vi "Channel Inputs.vi"(0 "Data Notifier":refnum<notifier>, 11 "error in":errorcluster={"status"=TRUE, "code"=0, "source"=""}) -> (3 "BangBang\nArm out":bool, 4 "Data Notifier out":refnum<notifier>, 6 "Actuation Array":bool[](array[boolean]), 10 "Auto-sequence":bool, 14 "Abort":bool, 15 "error out":errorcluster)   [LabVIEW 2024]
uses:
  78c51032-1941-47d2-9962-ba45e907be92.vi
  <vilib>/ErrorRing/Error Ring.xnode
  <vilib>/Utility/error.llb/Error Cluster From Error Code.vi
  support/Control/Array Data Constant.ctl
panel:
  in  "Prop Test":T1(array[cluster])=[{"Valve Label"="Fuel Iso", "Valve Index"=10, "Talkback Index"=9, "Actuate?"=TRUE, "Timeout"=10.0}, {"Valve Label"="LOX Iso", "Valve Index"=3, "Talkback Index"=3, "Actuate?"=TRUE, "Timeout"=10.0}, {"Valve Label"="Fuel Main", "Valve Index"=11, "Talkback Index"=10, "Actuate?"=TRUE, "Timeout"=10.0}, {"Valve Label"="LOX Main", "Valve Index"=4, "Talkback Index"=4, "Actuate?"=TRUE, "Timeout"=10.0}, {"Valve Label"="LOX Bleed", "Valve Index"=5, "Talkback Index"=5, "Actuate?"=TRUE, "Timeout"=10.0}]
  in  "NonProp Test":T1(array[cluster])=[{"Valve Label"="LOX Press", "Valve Index"=0, "Talkback Index"=0, "Actuate?"=TRUE, "Timeout"=24.0}, {"Valve Label"="Fuel Press", "Valve Index"=7, "Talkback Index"=6, "Actuate?"=TRUE, "Timeout"=24.0}, {"Valve Label"="LOX Vent", "Valve Index"=2, "Talkback Index"=2, "Actuate?"=TRUE, "Timeout"=4.0}, {"Valve Label"="Fuel Vent", "Valve Index"=9, "Talkback Index"=8, "Actuate?"=TRUE, "Timeout"=4.0}, {"Valve Label"="Fuel Purge", "Valve Index"=8, "Talkback Index"=7, "Actuate?"=TRUE, "Timeout"=2.0}, {"Valve Label"="LOX Purge", "Valve Index"=1, "Talkback Index"=1, "Actuate?"=TRUE, "Timeout"=2.0}, {"Valve Label"="Fuel Iso", "Valve Index"=10, "Talkback Index"=9, "Actuate?"=FALSE, "Timeout"=2.0}, {"Valve Label"="LOX Iso", "Valve Index"=3, "Talkback Index"=3, "Actuate?"=FALSE, "Timeout"=2.0}, {"Valve Label"="Fuel Main", "Valve Index"=11, "Talkback Index"=10, "Actuate?"=FALSE, "Timeout"=2.0}, {"Valve Label"="LOX Main", "Valve Index"=4, "Talkback Index"=4, "Actuate?"=FALSE, "Timeout"=2.0}, {"Valve Label"="LOX Bleed", "Valve Index"=5, "Talkback Index"=5, "Actuate?"=FALSE, "Timeout"=2.0}]
  in  "BangBang\nEnable":bool
  out "Time":dbl
  out "Actuate":bool caption="Should\nActuate?"
  out "LED 18":bool
  out "LED 17":bool
  out "LED 16":bool
  out "LED 15":bool
  out "LED 14":bool
  out "LED 13":bool
  out "LED 12":bool
  out "LED 11":bool
  out "LED 10":bool
  out "LED 9":bool
  out "LED 8":bool
  out "LED 7":bool
  out "LED 6":bool
  out "LED 5":bool
  out "LED 4":bool
  out "LED 3":bool
  out "LED 2":bool
  out "LED 1":bool
  out "Actuation Check":string
  in  "Actuation Check":bool caption="TC3\nActuation\nCheck"
  in  "Abort":bool
  in  "Switch 18":bool
  in  "Switch 17":bool
  in  "AutoSeq":bool
  in  "PropFlow":bool
  in  "Switch 16":bool
  in  "Switch 15":bool caption="LOX\nLoad"
  in  "Switch 14":bool caption="LOX\nBleed"
  in  "Switch 13":bool caption="LOX\nMain"
  in  "Switch 12":bool caption="LOX\nIso"
  in  "Switch 11":bool caption="LOX\nVent"
  in  "Switch 10":bool caption="LOX\nPurge"
  in  "Switch 9":bool caption="LOX\nPress"
  in  "Switch 8":bool
  in  "Switch 7":bool
  in  "Switch 6":bool
  in  "Switch 5":bool caption="Fuel\nMain"
  in  "Switch 4":bool caption="Fuel\nIso"
  in  "Switch 3":bool caption="Fuel\nVent"
  in  "Switch 2":bool caption="Fuel\nPurge"
  in  "Switch 1":bool caption="Fuel\nPress"
  in  "Software\nSwitch":bool
  out "Prop Flow":bool
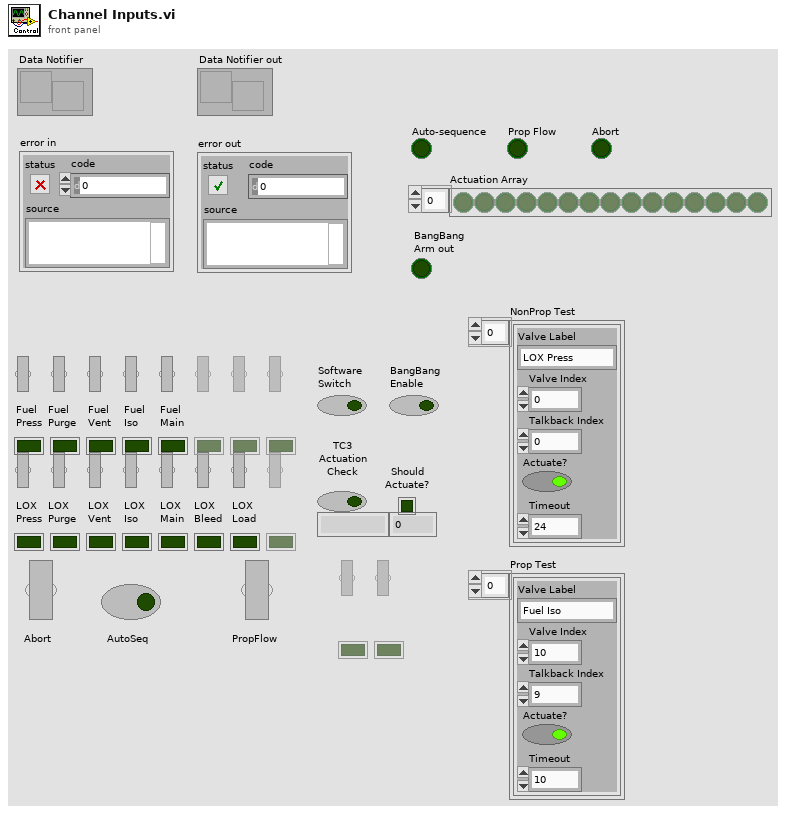
[diagram p1: front panel]
types:
  T1 = cluster{"Valve Label":string, "Valve Index":i32, "Talkback Index":i32, "Actuate?":bool, "Timeout":dbl}[]
  T2 = typedef "Array Data Constant.ctl" = cluster{"AI":dbl[], "TC":dbl[], "BC":dbl[], "DI":dbl[], "t (UTC)":dbl}
  T3 = cluster{"[0]":bool, "[1]":bool, "[2]":bool, "[3]":bool, "[4]":bool, "[5]":bool, "[6]":bool, "[7]":bool, "[8]":bool, "[9]":bool, "[10]":bool, "[11]":bool, "[12]":bool, "[13]":bool, "[14]":bool, "[15]":bool}
  T4 = cluster{"Valve Label":string, "Valve Index":i32, "Talkback Index":i32, "Actuate?":bool, "Timeout":dbl}
  T5 = cluster{"Switch 9":bool, "Switch 10":bool, "Switch 11":bool, bool, bool, bool, bool, "Switch 1":bool, "Switch 2":bool, "Switch 3":bool, bool, bool, bool, bool, bool, bool, bool, bool, bool, bool}
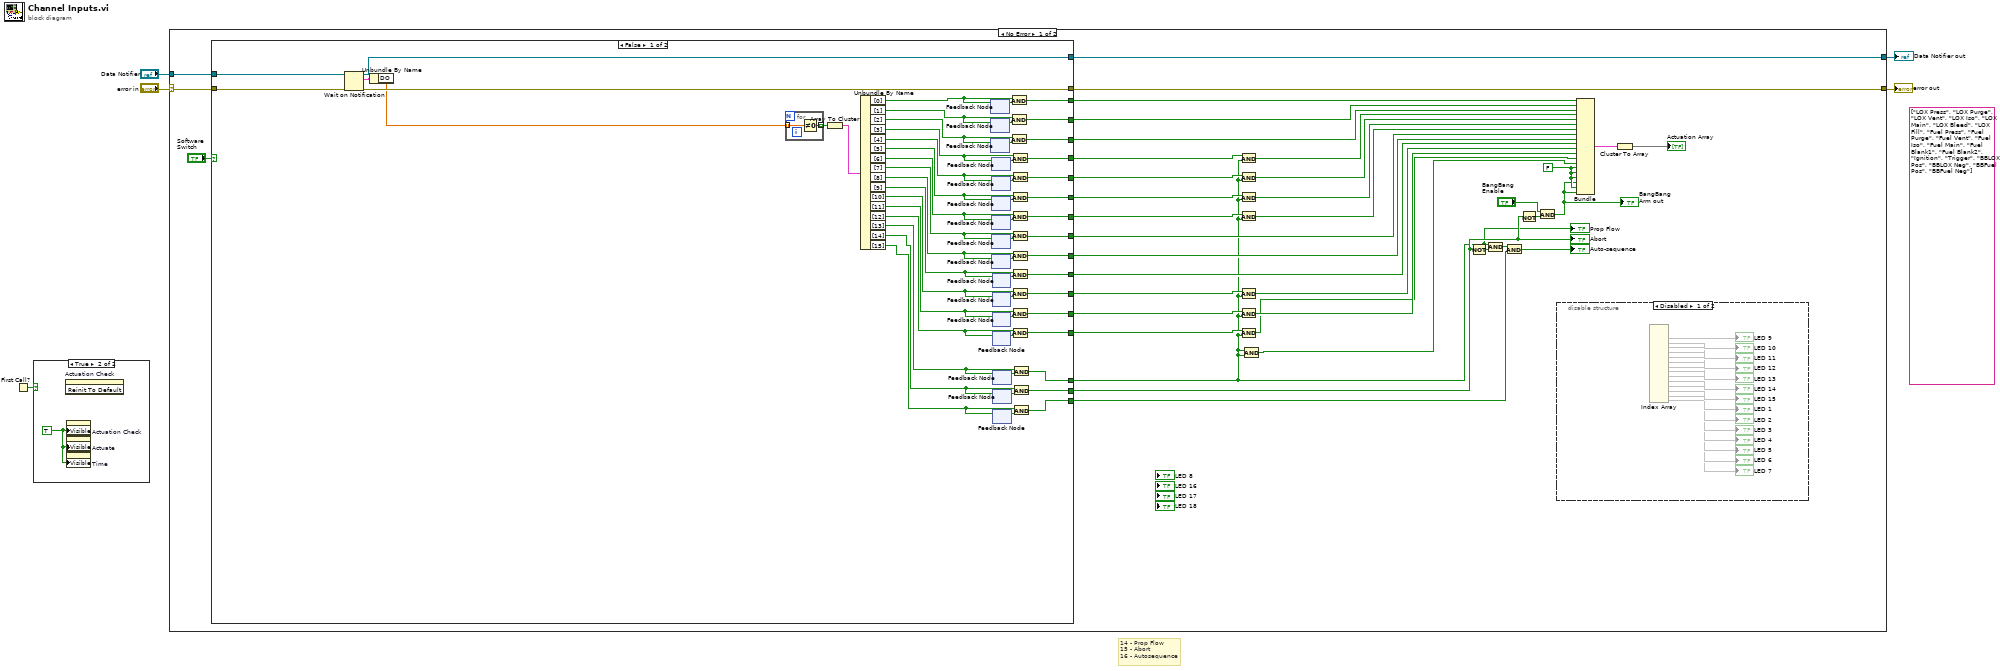
[diagram p0: block diagram]
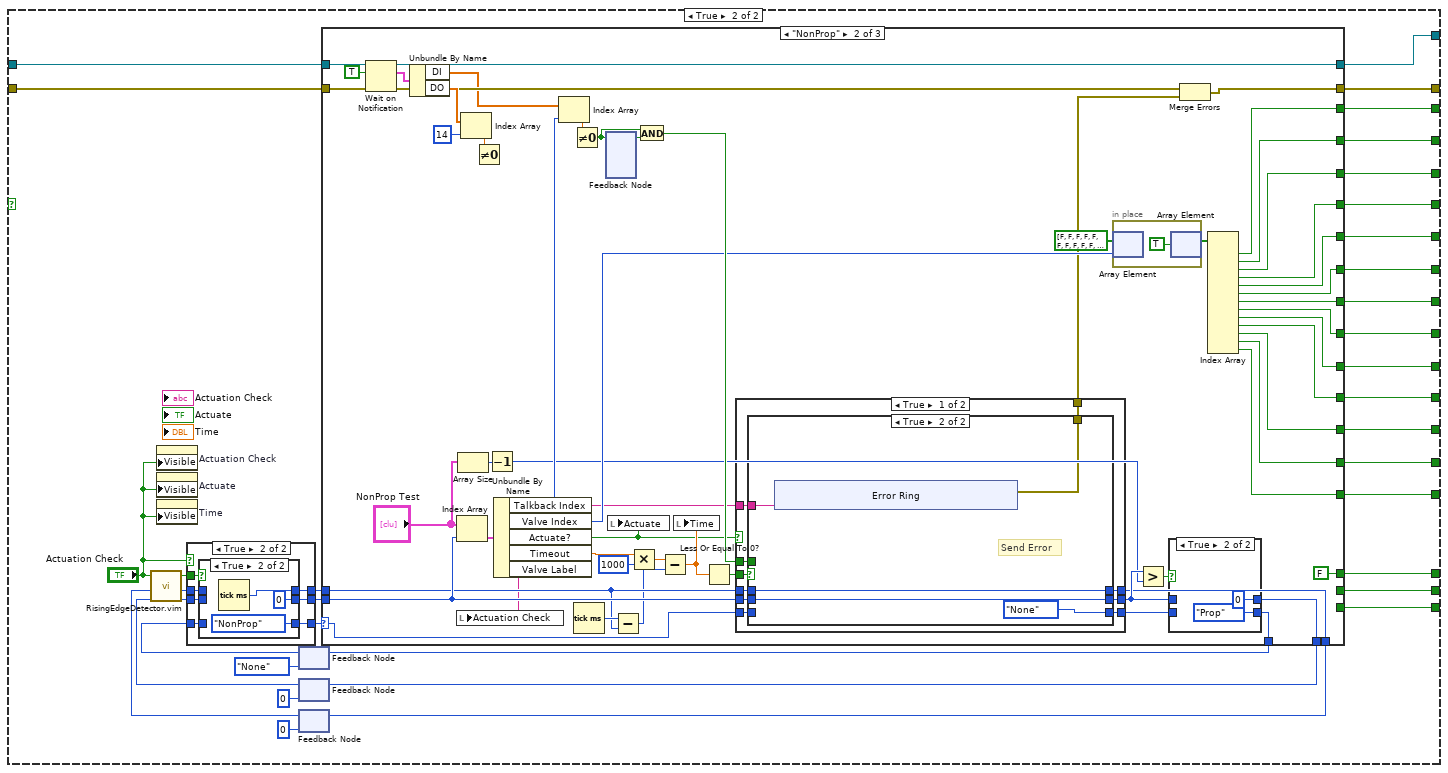
[diagram p4: hidden frame]
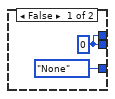
[diagram p5: hidden frame]
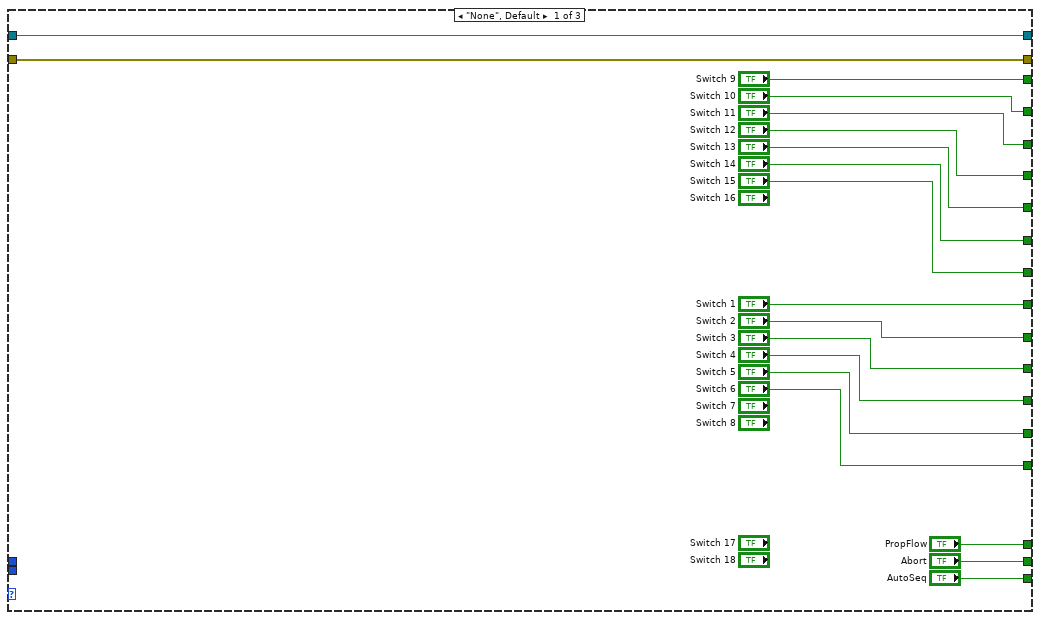
[diagram p7: hidden frame]
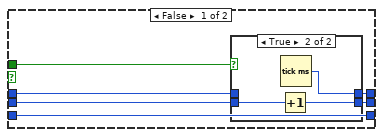
[diagram p9: hidden frame]
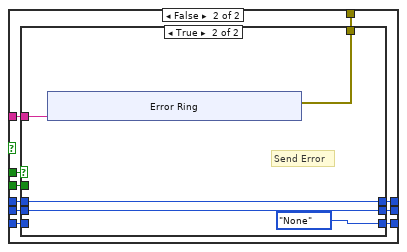
[diagram p11: hidden frame]
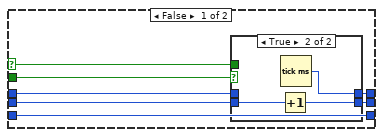
[diagram p12: hidden frame]
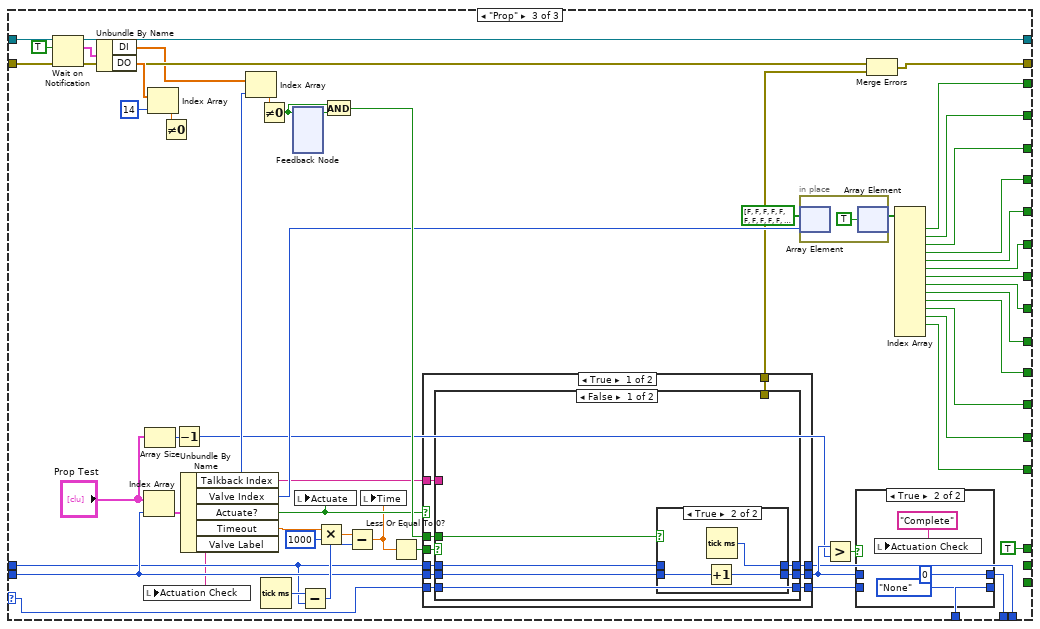
[diagram p14: hidden frame]
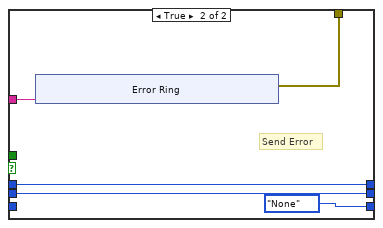
[diagram p17: hidden frame]
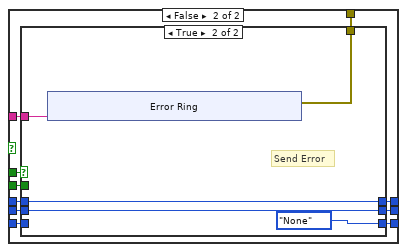
[diagram p18: hidden frame]
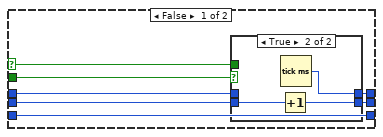
[diagram p19: hidden frame]
diagram:
  (unwired) string[] ["LOX Press", "LOX Purge", "LOX Vent", "LOX Iso", "LOX Main", "LOX Bleed", "LOX Fill", "Fuel Press", "Fuel Purge", "Fuel Vent", "Fuel Iso", "Fuel Main", "Fuel Blank1", "Fuel Blank2", "Ignition", "Trigger", "BBLOX Pos", "BBLOX Neg", "BBFuel Pos", "BBFuel Neg"]
  # "14 - Prop Flow\n15 - Abort\n16 - Autosequence"
  n1 = First Call?() -> (First Call?: T/F=w1:bool)
  n2 = case shown="True" w1 {
    frame False {
    }
    frame True {
      w6 = TRUE ("Visible")
      n3 = invoke on="Actuation Check" class="Bool (strict)" method="Reinit To Default"() -> ()  [unwired: 3 in, 3 out]
      n4 = property on="Actuation Check" class="Str"("Visible"=w6) -> ()  [unwired: 2 in, 2 out]
      n5 = property on="Actuate" class="Bool (strict)"("Visible"=w6) -> ()  [unwired: 2 in, 2 out]
      n6 = property on="Time" class="DigNum (strict)"("Visible"=w6) -> ()  [unwired: 2 in, 2 out]
    }
  }
  n7 = case shown="No Error" "error in" {
    selector: "error in" -> [w44 w442]
    tunnel: [w43 w442] -> w4
    tunnel: "Data Notifier" -> [w36 w441]
    tunnel: [w23 w441] -> w2
    frame No Error {
      w22 = FALSE
      n8 = case shown="False" "Software\nSwitch" {
        tunnel: w44 -> [w69 w124]
        tunnel: [w68 w123] -> w43
        tunnel: [w114 w149] -> w7
        tunnel: [w93 w148] -> w35
        tunnel: [w92 w141] -> w34
        tunnel: [w91 w140] -> w33
        tunnel: [w90 w139] -> w32
        tunnel: [w89 w138] -> w31
        tunnel: [w88 w137] -> w30
        tunnel: [w87 w150] -> w38
        tunnel: [w86 w135] -> w18
        tunnel: [w75 w136] -> w29
        tunnel: [w74 w147] -> w28
        tunnel: [w73 w146] -> w27
        tunnel: [w72 w145] -> w26
        tunnel: [w71 w144] -> w16
        tunnel: [w70 w143] -> w17
        tunnel: [w59 w142] -> w25
        tunnel: w36 -> [w67 w134]
        tunnel: [w66 w133] -> w23
        frame False {
          n9 = Wait on Notification(notifier=w67, error in (no error)=w69) -> (notifier out=w66:refnum<notifier>, notification=w65:T2, error out=w68:errorcluster)  [unwired: 2 in, 1 out]
          n10 = Unbundle By Name(w65) -> ("DO"=w64:dbl[])
          n11 = for {
            tunnel: w64 -> [w115] mode=indexing
            tunnel: [w116] -> w63 mode=indexing
            n12 = Not Equal To 0?(x=w115) -> (x != 0?=w116:bool)
          }
          n13 = Array To Cluster(array=w63) -> (cluster=w113:T3)
          n14 = Unbundle By Name(w113) -> ("[0]"=w96:bool, "[1]"=w95:bool, "[2]"=w94:bool, "[3]"=w85:bool, "[4]"=w84:bool, "[5]"=w83:bool, "[6]"=w82:bool, "[7]"=w81:bool, "[8]"=w80:bool, "[9]"=w79:bool, "[10]"=w78:bool, "[11]"=w77:bool, "[12]"=w76:bool, "[13]"=w62:bool, "[14]"=w61:bool, "[15]"=w60:bool)
          n15 = feedback #1() -> (w112:bool)  [unwired: 1 in]
          n16 = feedback-in #1(w96) -> ()
          n17 = feedback #2() -> (w111:bool)  [unwired: 1 in]
          n18 = feedback-in #2(w95) -> ()
          n19 = feedback #3() -> (w110:bool)  [unwired: 1 in]
          n20 = feedback-in #3(w94) -> ()
          n21 = feedback #4() -> (w109:bool)  [unwired: 1 in]
          n22 = feedback-in #4(w85) -> ()
          n23 = feedback #5() -> (w108:bool)  [unwired: 1 in]
          n24 = feedback-in #5(w84) -> ()
          n25 = feedback #6() -> (w107:bool)  [unwired: 1 in]
          n26 = feedback-in #6(w83) -> ()
          n27 = feedback #7() -> (w106:bool)  [unwired: 1 in]
          n28 = feedback-in #7(w82) -> ()
          n29 = feedback #8() -> (w105:bool)  [unwired: 1 in]
          n30 = feedback-in #8(w81) -> ()
          n31 = feedback #9() -> (w104:bool)  [unwired: 1 in]
          n32 = feedback-in #9(w80) -> ()
          n33 = feedback #10() -> (w103:bool)  [unwired: 1 in]
          n34 = feedback-in #10(w79) -> ()
          n35 = feedback #11() -> (w102:bool)  [unwired: 1 in]
          n36 = feedback-in #11(w78) -> ()
          n37 = feedback #12() -> (w101:bool)  [unwired: 1 in]
          n38 = feedback-in #12(w77) -> ()
          n39 = feedback #13() -> (w100:bool)  [unwired: 1 in]
          n40 = feedback-in #13(w76) -> ()
          n41 = feedback #14() -> (w99:bool)  [unwired: 1 in]
          n42 = feedback-in #14(w62) -> ()
          n43 = feedback #15() -> (w98:bool)  [unwired: 1 in]
          n44 = feedback-in #15(w61) -> ()
          n45 = feedback #16() -> (w97:bool)  [unwired: 1 in]
          n46 = feedback-in #16(w60) -> ()
          n47 = And(x=w96, y=w112) -> (x .and. y?=w93:bool)
          n48 = And(x=w95, y=w111) -> (x .and. y?=w92:bool)
          n49 = And(x=w94, y=w110) -> (x .and. y?=w91:bool)
          n50 = And(x=w85, y=w109) -> (x .and. y?=w90:bool)
          n51 = And(x=w84, y=w108) -> (x .and. y?=w89:bool)
          n52 = And(x=w83, y=w107) -> (x .and. y?=w88:bool)
          n53 = And(x=w82, y=w106) -> (x .and. y?=w75:bool)
          n54 = And(x=w81, y=w105) -> (x .and. y?=w74:bool)
          n55 = And(x=w80, y=w104) -> (x .and. y?=w73:bool)
          n56 = And(x=w79, y=w103) -> (x .and. y?=w72:bool)
          n57 = And(x=w78, y=w102) -> (x .and. y?=w71:bool)
          n58 = And(x=w77, y=w101) -> (x .and. y?=w70:bool)
          n59 = And(x=w76, y=w100) -> (x .and. y?=w59:bool)
          n60 = And(x=w62, y=w99) -> (x .and. y?=w114:bool)
          n61 = And(x=w61, y=w98) -> (x .and. y?=w86:bool)
          n62 = And(x=w60, y=w97) -> (x .and. y?=w87:bool)
        }
        frame True {
          n63 = call "RisingEdgeDetector.vim"("Data"="Actuation Check") -> ("Edge?"=w118:bool)  [unwired: 4 in]
          n64 = property on="Actuation Check" class="Str"("Visible"="Actuation Check") -> ()  [unwired: 2 in, 2 out]
          n65 = property on="Actuate" class="Bool (strict)"("Visible"="Actuation Check") -> ()  [unwired: 2 in, 2 out]
          n66 = property on="Time" class="DigNum (strict)"("Visible"="Actuation Check") -> ()  [unwired: 2 in, 2 out]
          n67 = feedback #17(enum16{"None", "NonProp", "Prop"}."None") -> (w131:enum16{"None", "NonProp", "Prop"})
          n68 = feedback #18(u8 0) -> (w127:u8)
          n69 = feedback #19(u32 0) -> (w121:u32)
          n70 = case shown="True" "Actuation Check" {
            tunnel: w131 -> [_ w159]
            tunnel: [enum16{"None", "NonProp", "Prop"}."None" w158] -> w130
            tunnel: w127 -> [_ w157]
            tunnel: [w151 w156] -> w126
            tunnel: w121 -> [_ w155]
            tunnel: [w151 w154] -> w119
            tunnel: w118 -> [_ w153]
            frame False {
              w151 = u8 0
            }
            frame True {
              n71 = case shown="True" w153 {
                tunnel: w159 -> [w162 _]
                tunnel: [w162 enum16{"None", "NonProp", "Prop"}."NonProp"] -> w158
                tunnel: w157 -> [w161 _]
                tunnel: [w161 u8 0] -> w156
                tunnel: [w160 w163] -> w154
                tunnel: w155 -> [w160 _]
                frame False {
                }
                frame True {
                  n72 = Tick Count (ms)() -> (millisecond timer value=w163:u32)
                }
              }
            }
          }
          n73 = case shown="\"NonProp\"" w130 {
            selector: w130 -> [_ w201 w328]
            tunnel: ["AutoSeq" _ _] -> w150
            tunnel: ["PropFlow" FALSE ("PropFlow") TRUE ("PropFlow")] -> w149
            tunnel: ["Switch 9" w227 w355] -> w148
            tunnel: ["Switch 1" w220 w348] -> w147
            tunnel: ["Switch 2" w219 w347] -> w146
            tunnel: ["Switch 3" w218 w346] -> w145
            tunnel: ["Switch 4" w217 w345] -> w144
            tunnel: ["Switch 5" w216 w344] -> w143
            tunnel: ["Switch 6" w215 w343] -> w142
            tunnel: ["Switch 10" w226 w354] -> w141
            tunnel: ["Switch 11" w225 w353] -> w140
            tunnel: ["Switch 12" w224 w352] -> w139
            tunnel: ["Switch 13" w223 w351] -> w138
            tunnel: ["Switch 14" w222 w350] -> w137
            tunnel: ["Switch 15" w221 w349] -> w136
            tunnel: ["Abort" _ _] -> w135
            tunnel: w134 -> [w168 w237 w365]
            tunnel: [w168 w235 w363] -> w133
            tunnel: [_ w196 w323] -> w129
            tunnel: [_ w194 w321] -> w128
            tunnel: w126 -> [_ w208 w335]
            tunnel: w124 -> [w167 w236 w364]
            tunnel: [w167 w203 w330] -> w123
            tunnel: [_ w192 w319] -> w120
            tunnel: w119 -> [_ w193 w320]
            frame "None", Default {
            }
            frame "NonProp" {
              n74 = Wait on Notification(notifier=w237, ignore previous (F)=TRUE, error in (no error)=w236) -> (notifier out=w235:refnum<notifier>, notification=w234:T2, error out=w204:errorcluster)  [unwired: 1 in, 1 out]
              n75 = Unbundle By Name(w234) -> ("DI"=w188:dbl[], "DO"=w230:dbl[])
              n76 = Index Array(array="NonProp Test", index=w208) -> (element=w239:T4)
              n77 = Array Size(array="NonProp Test") -> (size(s)=w199:i32)
              n78 = Index Array(array=w230, index=14) -> (element=w229:dbl)
              n79 = Not Equal To 0?(x=w229) -> ()  [unwired: 1 out]
              n80 = Decrement(x=w199) -> (x-1=w190:i32)
              n81 = Unbundle By Name(w239) -> ("Talkback Index"=w212:i32, "Valve Index"=w205:i32, "Actuate?"=w184:bool, "Timeout"=w210:dbl, "Valve Label"=w189:string)
              n82 = local write "Actuation Check"(w189) -> ()
              n83 = Index Array(array=w188, index=w212) -> (element=w228:dbl)
              n84 = Not Equal To 0?(x=w228) -> (x != 0?=w232:bool)
              n85 = Tick Count (ms)() -> (millisecond timer value=w209:u32)
              n86 = feedback-in #20(w232) -> ()
              n87 = feedback #20() -> (w233:bool)  [unwired: 1 in]
              n88 = local write "Actuate"(w184) -> ()
              n89 = Subtract(x=w209, y=w193) -> (x-y=w187:u32)
              n90 = Multiply(x=w210, y=u32 1000 ("x")) -> (x*y=w186:dbl)
              n91 = And(x=w232, y=w233) -> (x .and. y?=w206:bool)
              n92 = Subtract(x=w186, y=w187) -> (x-y=w185:dbl)
              n93 = local write "Time"(w185) -> ()
              n94 = Less Or Equal To 0?(x=w185) -> (x <= 0?=w207:bool)
              n95 = case shown="True" w184 {
                tunnel: w208 -> [w252 w285]
                tunnel: [w251 w284] -> w195
                tunnel: w207 -> [w253 w286]
                tunnel: w206 -> [w250 w283]
                tunnel: [w249 w282] -> w202
                tunnel: [w248 w281] -> w197
                tunnel: w201 -> [w247 w280]
                tunnel: w193 -> [w246 w279]
                tunnel: [w245 w278] -> w192
                tunnel: w189 -> [w244 w277]
                frame True {
                  n96 = case shown="True" w253 {
                    tunnel: w252 -> [w258 w269]
                    tunnel: [w257 w269] -> w251
                    tunnel: w250 -> [w259 _]
                    tunnel: [_ w266] -> w249
                    tunnel: [w256 enum16{"None", "NonProp", "Prop"}."None"] -> w248
                    tunnel: w247 -> [w256 _]
                    tunnel: w246 -> [w255 w267]
                    tunnel: [w254 w267] -> w245
                    tunnel: w244 -> [_ w265]
                    frame False {
                      n97 = case shown="True" w259 {
                        tunnel: w258 -> [w261 w264]
                        tunnel: [w261 w263] -> w257
                        tunnel: w255 -> [w260 _]
                        tunnel: [w260 w262] -> w254
                        frame False {
                        }
                        frame True {
                          n98 = Increment(x=w264) -> (x+1=w263:u8)
                          n99 = Tick Count (ms)() -> (millisecond timer value=w262:u32)
                        }
                      }
                    }
                    frame True {
                      # "Send Error"
                      n100 = xnode "Error Ring"("parameter 0"=w265) -> ("error out"=w266:errorcluster)
                    }
                  }
                }
                frame False {
                  n101 = case shown="True" w283 {
                    selector: w283 -> [w293 _]
                    tunnel: w285 -> [w292 w303]
                    tunnel: [w291 w303] -> w284
                    tunnel: [_ w300] -> w282
                    tunnel: [w290 enum16{"None", "NonProp", "Prop"}."None"] -> w281
                    tunnel: w280 -> [w290 _]
                    tunnel: w286 -> [w289 _]
                    tunnel: w279 -> [w288 w301]
                    tunnel: [w287 w301] -> w278
                    tunnel: w277 -> [_ w299]
                    frame False {
                      n102 = case shown="True" w289 {
                        tunnel: w292 -> [w295 w298]
                        tunnel: [w295 w297] -> w291
                        tunnel: w293 -> [_ _]
                        tunnel: w288 -> [w294 _]
                        tunnel: [w294 w296] -> w287
                        frame False {
                        }
                        frame True {
                          n103 = Increment(x=w298) -> (x+1=w297:u8)
                          n104 = Tick Count (ms)() -> (millisecond timer value=w296:u32)
                        }
                      }
                    }
                    frame True {
                      # "Send Error"
                      n105 = xnode "Error Ring"("parameter 0"=w299) -> ("error out"=w300:errorcluster)
                    }
                  }
                }
              }
              n106 = in-place {
                n107 = in-place-array #21(bool[] [FALSE, FALSE, FALSE, FALSE, FALSE, FALSE, FALSE, FALSE, FALSE, FALSE, FALSE, FALSE, FALSE, FALSE, FALSE, FALSE, FALSE, FALSE, FALSE, FALSE, FALSE], w205) -> ()  [unwired: 1 out]
                n108 = in-place-array #21(TRUE ("element")) -> (w213:bool[])  [unwired: 1 out]
              }
              n109 = Greater?(x=w195, y=w190) -> (0:w198:bool)
              n110 = case shown="True" w198 {
                tunnel: w197 -> [w240 _]
                tunnel: [w240 enum16{"None", "NonProp", "Prop"}."Prop"] -> w196
                tunnel: w195 -> [w241 _]
                tunnel: [w241 u8 0] -> w194
                frame False {
                }
                frame True {
                }
              }
              n111 = Merge Errors(w204, w202) -> (w203:errorcluster)
              n112 = Index Array(array=w213) -> (element #1=w227:bool, element #2=w226:bool, element #3=w225:bool, element #4=w224:bool, element #5=w223:bool, element #6=w222:bool, element #7=w221:bool, element #8=w220:bool, element #9=w219:bool, element #10=w218:bool, element #11=w217:bool, element #12=w216:bool, element #13=w215:bool)  [unwired: 13 in]
            }
            frame "Prop" {
              n113 = Wait on Notification(notifier=w365, ignore previous (F)=TRUE, error in (no error)=w364) -> (notifier out=w363:refnum<notifier>, notification=w362:T2, error out=w331:errorcluster)  [unwired: 1 in, 1 out]
              n114 = Unbundle By Name(w362) -> ("DI"=w315:dbl[], "DO"=w358:dbl[])
              n115 = Index Array(array="Prop Test", index=w335) -> (element=w367:T4)
              n116 = Array Size(array="Prop Test") -> (size(s)=w326:i32)
              n117 = Index Array(array=w358, index=14) -> (element=w357:dbl)
              n118 = Not Equal To 0?(x=w357) -> ()  [unwired: 1 out]
              n119 = Decrement(x=w326) -> (x-1=w317:i32)
              n120 = Unbundle By Name(w367) -> ("Talkback Index"=w340:i32, "Valve Index"=w332:i32, "Actuate?"=w314:bool, "Timeout"=w338:dbl, "Valve Label"=w316:string)
              n121 = local write "Actuation Check"(w316) -> ()
              n122 = Index Array(array=w315, index=w340) -> (element=w356:dbl)
              n123 = Not Equal To 0?(x=w356) -> (x != 0?=w360:bool)
              n124 = Tick Count (ms)() -> (millisecond timer value=w337:u32)
              n125 = feedback-in #22(w360) -> ()
              n126 = feedback #22() -> (w361:bool)  [unwired: 1 in]
              n127 = local write "Actuate"(w314) -> ()
              n128 = Subtract(x=w337, y=w320) -> (x-y=w336:u32)
              n129 = Multiply(x=w338, y=u32 1000 ("x")) -> (x*y=w313:dbl)
              n130 = And(x=w360, y=w361) -> (x .and. y?=w333:bool)
              n131 = Subtract(x=w313, y=w336) -> (x-y=w312:dbl)
              n132 = local write "Time"(w312) -> ()
              n133 = Less Or Equal To 0?(x=w312) -> (x <= 0?=w334:bool)
              n134 = case shown="True" w314 {
                tunnel: w335 -> [w381 w414]
                tunnel: [w380 w413] -> w322
                tunnel: w334 -> [w382 w415]
                tunnel: w333 -> [w379 w412]
                tunnel: [w378 w411] -> w329
                tunnel: [w377 w410] -> w324
                tunnel: w328 -> [w376 w409]
                tunnel: w320 -> [w375 w408]
                tunnel: [w374 w407] -> w319
                tunnel: w316 -> [w373 w406]
                frame True {
                  n135 = case shown="False" w382 {
                    tunnel: w381 -> [w387 w398]
                    tunnel: [w386 w398] -> w380
                    tunnel: w379 -> [w388 _]
                    tunnel: [_ w395] -> w378
                    tunnel: [w385 enum16{"None", "NonProp", "Prop"}."None"] -> w377
                    tunnel: w376 -> [w385 _]
                    tunnel: w375 -> [w384 w396]
                    tunnel: [w383 w396] -> w374
                    tunnel: w373 -> [_ w394]
                    frame False {
                      n136 = case shown="True" w388 {
                        tunnel: w387 -> [w390 w393]
                        tunnel: [w390 w392] -> w386
                        tunnel: w384 -> [w389 _]
                        tunnel: [w389 w391] -> w383
                        frame False {
                        }
                        frame True {
                          n137 = Increment(x=w393) -> (x+1=w392:u8)
                          n138 = Tick Count (ms)() -> (millisecond timer value=w391:u32)
                        }
                      }
                    }
                    frame True {
                      # "Send Error"
                      n139 = xnode "Error Ring"("parameter 0"=w394) -> ("error out"=w395:errorcluster)
                    }
                  }
                }
                frame False {
                  n140 = case shown="True" w412 {
                    selector: w412 -> [w422 _]
                    tunnel: w414 -> [w421 w432]
                    tunnel: [w420 w432] -> w413
                    tunnel: [_ w429] -> w411
                    tunnel: [w419 enum16{"None", "NonProp", "Prop"}."None"] -> w410
                    tunnel: w409 -> [w419 _]
                    tunnel: w415 -> [w418 _]
                    tunnel: w408 -> [w417 w430]
                    tunnel: [w416 w430] -> w407
                    tunnel: w406 -> [_ w428]
                    frame False {
                      n141 = case shown="True" w418 {
                        tunnel: w421 -> [w424 w427]
                        tunnel: [w424 w426] -> w420
                        tunnel: w422 -> [_ _]
                        tunnel: w417 -> [w423 _]
                        tunnel: [w423 w425] -> w416
                        frame False {
                        }
                        frame True {
                          n142 = Increment(x=w427) -> (x+1=w426:u8)
                          n143 = Tick Count (ms)() -> (millisecond timer value=w425:u32)
                        }
                      }
                    }
                    frame True {
                      # "Send Error"
                      n144 = xnode "Error Ring"("parameter 0"=w428) -> ("error out"=w429:errorcluster)
                    }
                  }
                }
              }
              n145 = in-place {
                n146 = in-place-array #23(bool[] [FALSE, FALSE, FALSE, FALSE, FALSE, FALSE, FALSE, FALSE, FALSE, FALSE, FALSE, FALSE, FALSE, FALSE, FALSE, FALSE, FALSE, FALSE, FALSE, FALSE, FALSE], w332) -> ()  [unwired: 1 out]
                n147 = in-place-array #23(TRUE ("element")) -> (w341:bool[])  [unwired: 1 out]
              }
              n148 = Greater?(x=w322, y=w317) -> (0:w325:bool)
              n149 = case shown="True" w325 {
                tunnel: w324 -> [w368 _]
                tunnel: [w368 enum16{"None", "NonProp", "Prop"}."None"] -> w323
                tunnel: w322 -> [w369 _]
                tunnel: [w369 u8 0] -> w321
                frame False {
                }
                frame True {
                  n150 = local write "Actuation Check"("Complete") -> ()
                }
              }
              n151 = Merge Errors(w331, w329) -> (w330:errorcluster)
              n152 = Index Array(array=w341) -> (element #1=w355:bool, element #2=w354:bool, element #3=w353:bool, element #4=w352:bool, element #5=w351:bool, element #6=w350:bool, element #7=w349:bool, element #8=w348:bool, element #9=w347:bool, element #10=w346:bool, element #11=w345:bool, element #12=w344:bool, element #13=w343:bool)  [unwired: 14 in, 1 out]
            }
          }
          n153 = feedback-in #17(w129) -> ()
          n154 = feedback-in #18(w128) -> ()
          n155 = feedback-in #19(w120) -> ()
        }
      }
      "Prop Flow" <- w7
      "Abort" <- w18
      n156 = And(x=w32, y=w7) -> (x .and. y?=w15:bool)
      n157 = And(x=w31, y=w7) -> (x .and. y?=w14:bool)
      n158 = And(x=w30, y=w7) -> (x .and. y?=w13:bool)
      n159 = And(x=w29, y=w7) -> (x .and. y?=w10:bool)
      n160 = And(x=w16, y=w7) -> (x .and. y?=w12:bool)
      n161 = And(x=w17, y=w7) -> (x .and. y?=w11:bool)
      n162 = And(x=w25, y=w7) -> (x .and. y?=w9:bool)
      n163 = And(x=w7, y=w7) -> (x .and. y?=w8:bool)
      n164 = Not(x=w18) -> (.not. x?=w39:bool)
      n165 = And(x=w7, y=w39) -> (x .and. y?=w40:bool)
      n166 = And(x=w40, y=w38) -> (x .and. y?=→"Auto-sequence":bool)
      n167 = Not(x=w18) -> (.not. x?=w21:bool)
      n168 = And(x="BangBang\nEnable", y=w21) -> (x .and. y?=w19:bool)
      "BangBang\nArm out" <- w19
      n169 = disable-structure shown="Disabled" {
        frame Disabled {
          n170 = Index Array() -> (element #1=→"LED 9", element #2=→"LED 10", element #3=→"LED 11", element #4=→"LED 12", element #5=→"LED 13", element #6=→"LED 14", element #7=→"LED 15", element #8=→"LED 1", element #9=→"LED 2", element #10=→"LED 3", element #11=→"LED 4", element #12=→"LED 5", element #13=→"LED 6", element #14=→"LED 7")  [unwired: 15 in]
        }
        frame Enabled {
        }
      }
      n171 = Bundle("Switch 9"=w35, "Switch 10"=w34, "Switch 11"=w33, w15, w14, w13, w10, "Switch 1"=w28, "Switch 2"=w27, "Switch 3"=w26, w12, w11, w9, w8, w22, w22, w22, w19, w22, w19) -> (w41:T5)  [unwired: 1 in]
      n172 = Cluster To Array(cluster=w41) -> (array=→"Actuation Array":bool[])
    }
    frame Error {
    }
  }
  "error out" <- w4
  "Data Notifier out" <- w2
